vi "Initialize Active Routes.vi"(8 "error in (no error)":errorcluster, 11 "2525 in":refnum<class "2525.lvclass">) -> (0 "error out":errorcluster, 3 "2525 out":refnum<class "2525.lvclass">)   [LabVIEW 2019, in "2525.lvlib" / "2525.lvclass"]
uses:
  Library/2525.lvclass
  Library/2525.lvclass/2525.ctl
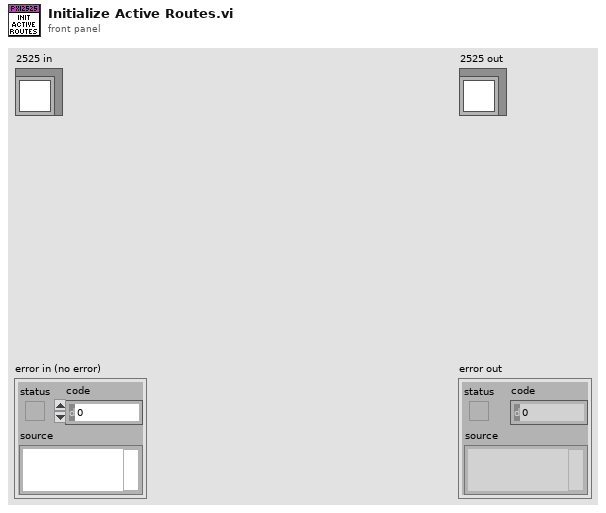
[diagram p1: front panel]
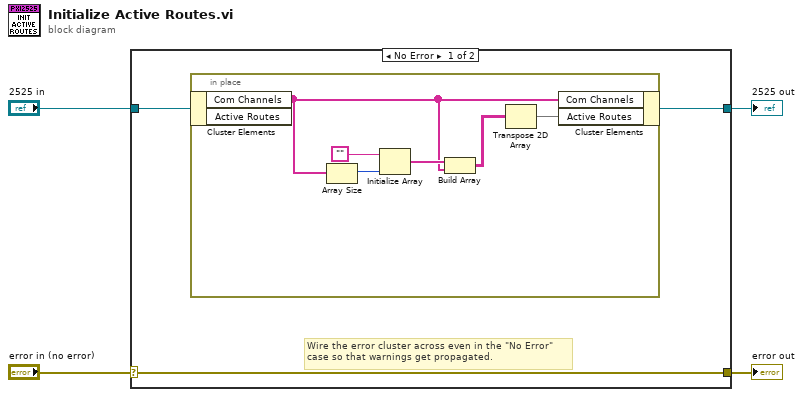
[diagram p0: block diagram]
diagram:
  n1 = case shown="No Error" "error in (no error)" {
    selector: "error in (no error)" -> [w7 w15]
    tunnel: [w7 w15] -> w3
    tunnel: [w5 w14] -> w1
    tunnel: "2525 in" -> [w6 w14]
    frame No Error {
      # "Wire the error cluster across even in the \"No Error\"\ncase so that warnings get propagated."
      n2 = in-place {
        n3 = in-place-cluster #1(w6) -> ("Com Channels"=w10:string[])  [unwired: 1 out]
        n4 = Array Size(array=w10) -> (size(s)=w13:i32)
        n5 = Initialize Array("", w13) -> (w11:string[])
        n6 = Build Array(w11, w10) -> (w9:string[][])
        n7 = Transpose 2D Array(2D array=w9) -> (transposed array=w8:string[][])
        n8 = in-place-cluster #1("Com Channels"=w10, "Active Routes"=w8) -> (w5:refnum<class "2525.lvclass">)
      }
    }
    frame Error {
    }
  }
  "error out" <- w3
  "2525 out" <- w1
